vi "Teleop.vi"(10 "Match Info":T1={"Autonomous Elapsed Seconds"=0.0, "TeleOp Elapsed Seconds"=0.0, "Disabled Elapsed Seconds"=0.0, "Visited Autonomous"=FALSE, "Visited TeleOp"=FALSE, "Visited Disabled"=FALSE, "Autonomous Settings"={"Autonomous Style"=enum."Independent", "VI Refnum"=refnum}}, 11 "Call Context":T2) -> ()   [LabVIEW 2015]
doc: "This VI is called for each TeleOp packet received from the DS where the robot is not disabled. It is often used to read from the joysticks and update I/O or to update setpoints for timed control loops. It should complete and return within 20 milliseconds or it may miss DS packets."
uses:
  <vilib>/Rock Robotics/WPI/DriverStation/WPI_DriverStationDerivedRobotMode.ctl
  <vilib>/Rock Robotics/WPI/DriverStation/WPI_DriverStationMatch Info.ctl
  <vilib>/Rock Robotics/WPI/Solenoid/WPI_SolenoidValue.ctl
  <vilib>/Rock Robotics/Network Tables/NT Read Boolean.vi
  <vilib>/Rock Robotics/Network Tables/NT Read Number.vi
  <vilib>/Rock Robotics/WPI/Utilities/WPI_GetSetVariantRefNum.vi
  <vilib>/Rock Robotics/WPI/Solenoid/WPI_SolenoidSetEnum.vi
  <vilib>/addons/control/pid/NI_PID_pid.lvlib
  <vilib>/addons/control/pid/pid.llb/PID (DBL).vi
panel:
  in  "Numeric":dbl
  out "Encodeur gauche min":dbl
  out "Encodeur gauche max":dbl
  out "Encodeur droit max":dbl
  out "Encodeur droit min":dbl
  out "Sample Slider 0":dbl(slide) scale=0.0..5.0
  out "Sample Boolean 1":bool
  out "Sample Boolean 0":bool
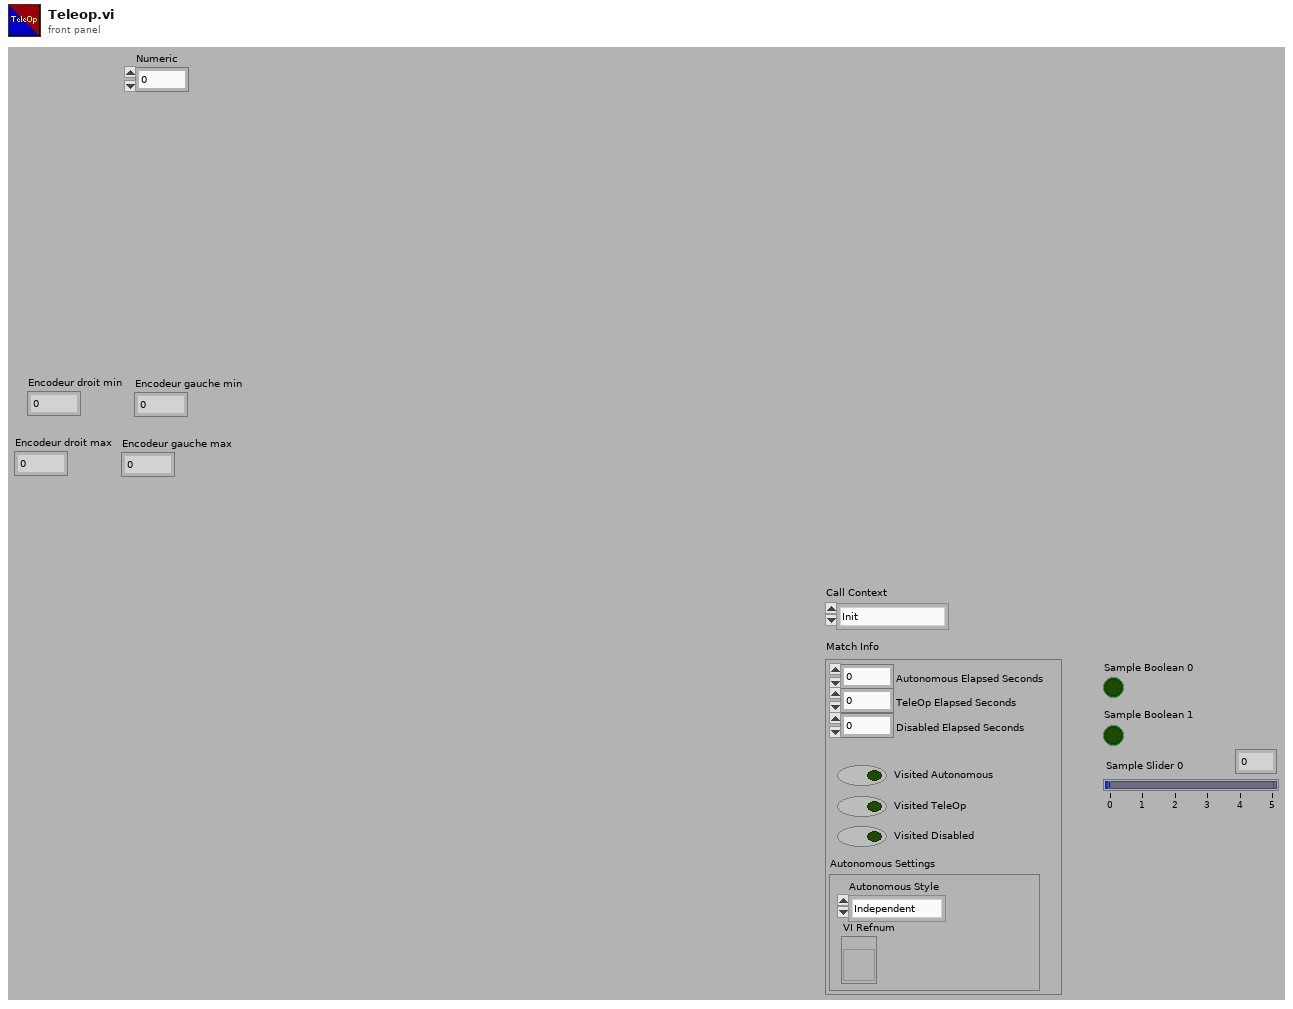
[diagram p1: front panel]
types:
  T1 = typedef "WPI_DriverStationMatch Info.ctl" = cluster{"Autonomous Elapsed Seconds":dbl, "TeleOp Elapsed Seconds":dbl, "Disabled Elapsed Seconds":dbl, "Visited Autonomous":bool, "Visited TeleOp":bool, "Visited Disabled":bool, "Autonomous Settings":cluster{"Autonomous Style":enum16{"Iterative", "Independent"}, "VI Refnum":refnum<vi>}}
  T2 = typedef "WPI_DriverStationDerivedRobotMode.ctl" = enum16{"Init", "Execute", "Stop"}
  T3 = typedef "WPI_JoystickDevRef.ctl" = cluster{"Device":T4}
  T4 = typedef "WPI_JoystickDeviceEnum.ctl" = enum16{"USB 0", "USB 1", "USB 2", "USB 3", "USB 4", "USB 5"}
  T5 = cluster{"Axes[0]":dbl, "Axes[1]":dbl, "Axes[2]":dbl, "Axes[3]":dbl, "Axes[4]":dbl, "Axes[5]":dbl, "Axes[6]":dbl, "Axes[7]":dbl, "Axes[8]":dbl}
  T6 = cluster{"Buttons[0]":bool, "Buttons[1]":bool, "Buttons[2]":bool, "Buttons[3]":bool, "Buttons[4]":bool, "Buttons[5]":bool, "Buttons[6]":bool, "Buttons[7]":bool, "Buttons[8]":bool}
  T7 = typedef "WPI_EncoderDevRef.ctl" = cluster{"DevStatus":errorcluster, "EncoderIndex":T8, "CounterIndex":T9, "DistancePerCount":dbl, "Decoding Type":T10}
  T8 = typedef "FPGA_EncoderIdx.ctl" = enum8{"Enc 0", "Enc 1", "Enc 2", "Enc 3", "Enc 4", "Enc 5", "Enc 6", "Enc 7", "Invalid"}
  T9 = typedef "FPGA_CounterCtrSystemIndex.ctl" = enum8{"Ctr 0", "Ctr 1", "Ctr 2", "Ctr 3", "Ctr 4", "Ctr 5", "Ctr 6", "Ctr 7", "Invalid"}
  T10 = typedef "WPI_EncoderType.ctl" = enum16{"1x", "2x", "4x"}
  T11 = cluster{"proportional gain (Kc)":dbl, "integral time (Ti, min)":dbl, "derivative time (Td, min)":dbl}
  T12 = typedef "WPI_SolenoidDevRef.ctl" = cluster{"DevStatus":errorcluster, "Pneumatics Control Module":u8, "Forward Solenoid Channel":T13, "Reverse Solenoid Channel":T13}
  T13 = typedef "WPI_SolenoidChannel.ctl" = enum8{"Solenoid 0", "Solenoid 1", "Solenoid 2", "Solenoid 3", "Solenoid 4", "Solenoid 5", "Solenoid 6", "Solenoid 7", "Invalid"}
  T14 = typedef "WPI_SolenoidValue.ctl" = enum16{"Off", "On", "Forward", "Reverse"}
  T15 = typedef "WPI_MotorControlDeviceRef.ctl" = cluster{"DeviceStatus":errorcluster, "Type":T16, "PWM":cluster{"PWM Channel":T17, "DeadBand":T18}, "CAN":cluster{"Device Number":u8, "Control Mode":T19, "Semaphore":T20, "Max Vout":dbl, "TalonSRX Control Mode":T21}, "Invert":bool}
  T16 = typedef "WPI_MotorControlType.ctl" = enum16{"PWM", "CAN", "CANTalonSRX"}
  T17 = typedef "FPGA_DIOPWMChannel.ctl" = enum8{"PWM 0", "PWM 1", "PWM 2", "PWM 3", "PWM 4", "PWM 5", "PWM 6", "PWM 7", "PWM 8", "PWM 9", "PWM MXP 0", "PWM MXP 1", "PWM MXP 2", "PWM MXP 3", "PWM MXP 4", "PWM MXP 5", "PWM MXP 6", "PWM MXP 7", "PWM MXP 8", "PWM MXP 9", "Invalid"}
  T18 = typedef "WPI_PWMDeadband.ctl" = cluster{"Name":string, "maxPositivePwm":i32, "minPositivePwm":i32, "centerPwm":i32, "maxNegativePwm":i32, "minNegativePwm":i32, "angularRange":u16}
  T19 = typedef "WPI_CANJaguar_ControlMode.ctl" = enum8{"Percent VBus", "Current", "Speed", "Position", "Voltage"}
  T20 = typedef "Semaphore RefNum" = refnum<k1>
  T21 = typedef "WPI_CANTalonSRX_APIControlMode.ctl" = enum8{"Percent VBus", "Speed", "Position", "Slave", "Unchanged / Invalid", "Voltage Compensation", "Current", "Motion Profile"}
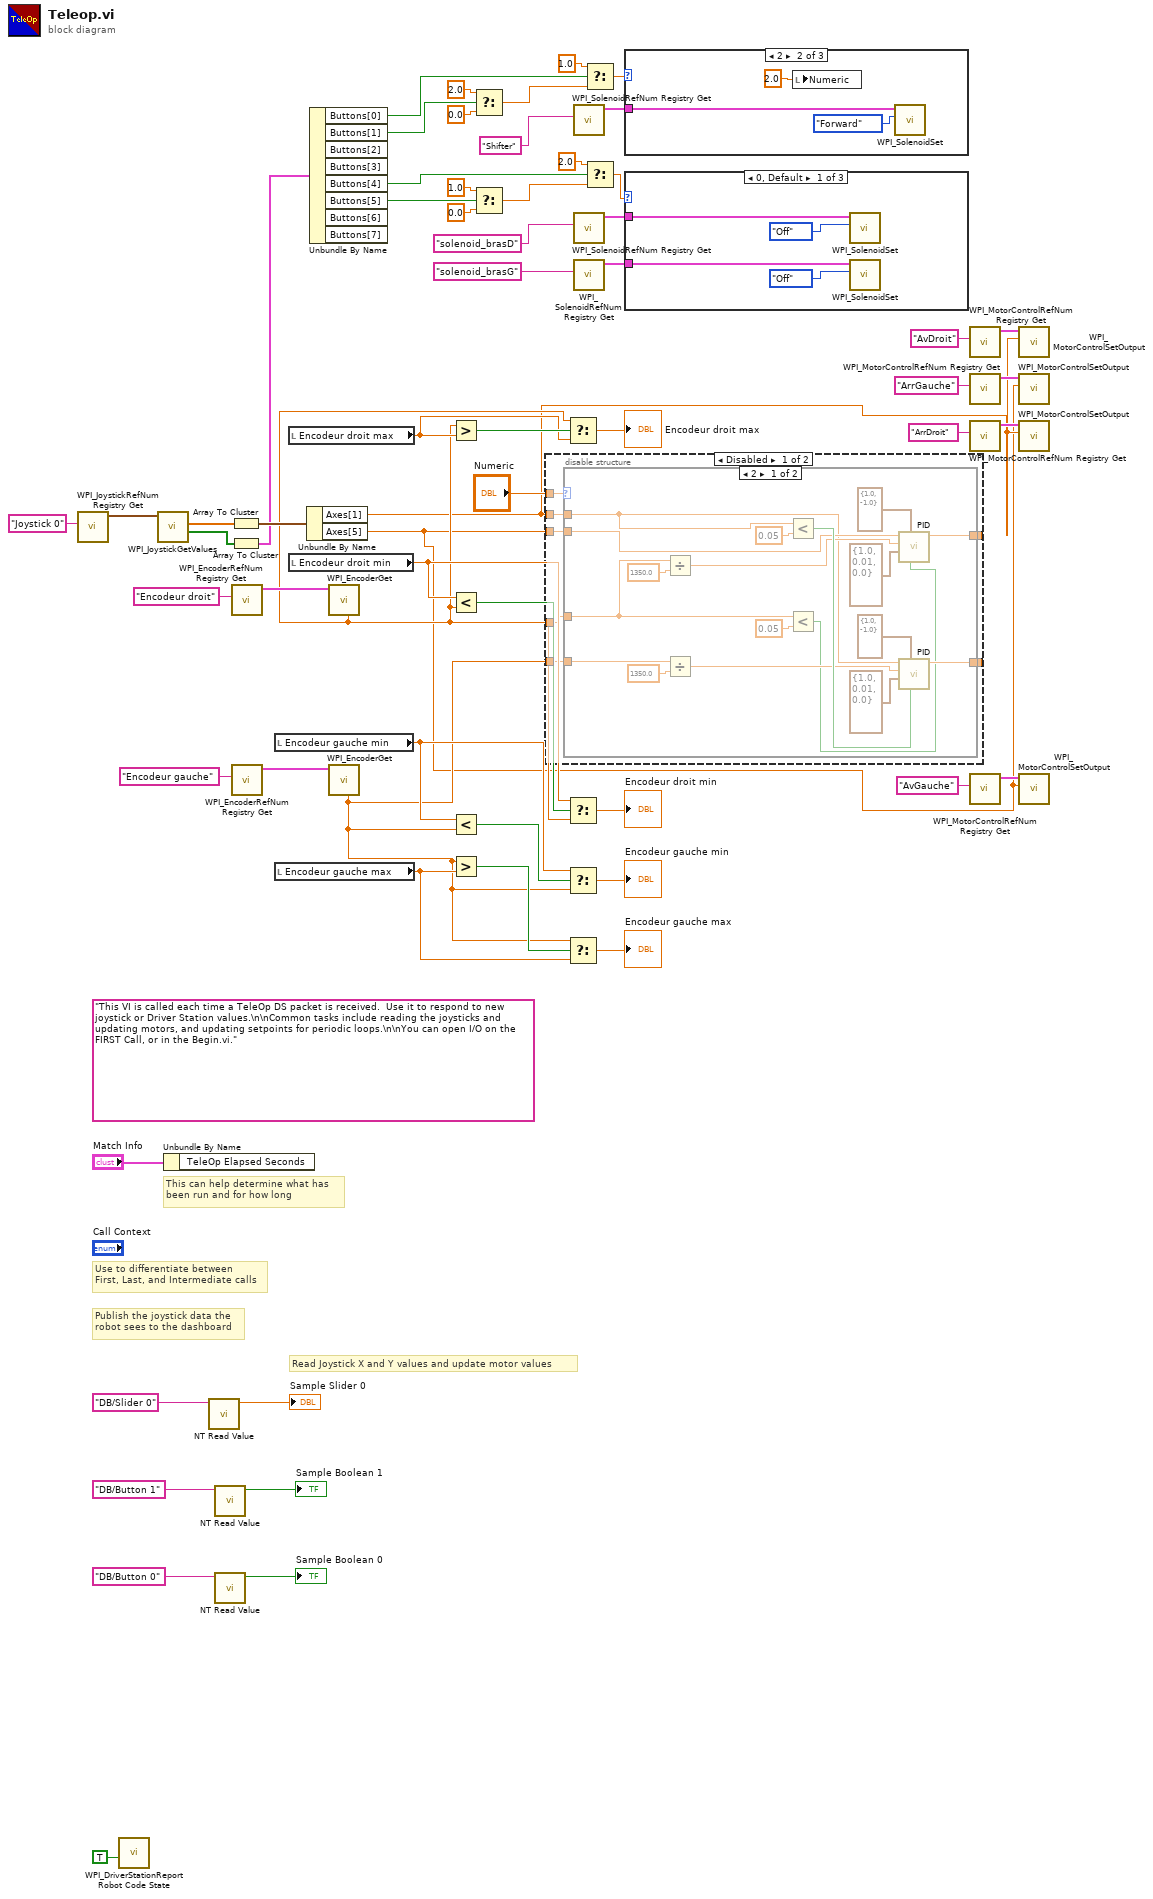
[diagram p0: block diagram]
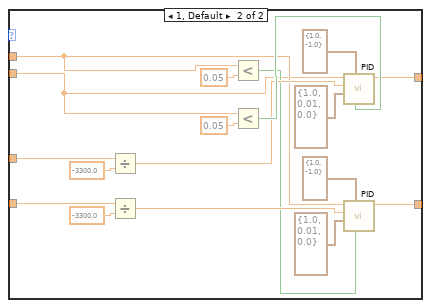
[diagram p2: hidden frame]
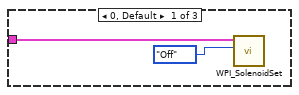
[diagram p4: hidden frame]
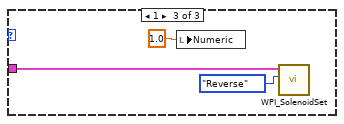
[diagram p5: hidden frame]
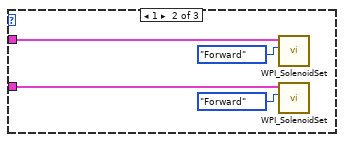
[diagram p6: hidden frame]
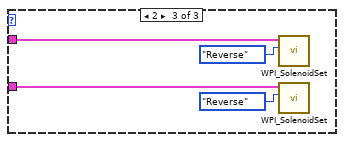
[diagram p7: hidden frame]
diagram:
  (unwired) "This VI is called each time a TeleOp DS packet is received.  Use it to respond to new joystick or Driver Station values.\n\nCommon tasks include reading the joysticks and updating motors, and updating setpoints for periodic loops.\n\nYou can open I/O on the FIRST Call, or in the Begin.vi."
  # "Publish the joystick data the\nrobot sees to the dashboard"
  # "Use to differentiate between\nFirst, Last, and Intermediate calls"
  # "This can help determine what has\nbeen run and for how long"
  # "Read Joystick X and Y values and update motor values"
  n1 = call <vilib>:"WPI_JoystickRefNum Registry Get.vi"("refnum name"="Joystick 0") -> ("JoystickDevRef"=w54:T3)  [unwired: 1 in, 9 out]
  n2 = call <vilib>:"WPI_DriverStationReport Robot Code State.vi"("TeleOp"=TRUE ("Autonomous")) -> ()  [unwired: 10 in, 1 out]
  n3 = call <vilib>:"WPI_JoystickGetValues.vi"("JoystickDevRef"=w54) -> ("Buttons"=w51:bool[], "Axes"=w53:dbl[])  [unwired: 6 in, 3 out]
  n4 = Unbundle By Name("Match Info") -> ()  [unwired: 1 out]
  n5 = call-poly <vilib>:"NT Read Value.vi"("Name"="DB/Slider 0" ("refnum name")) -> ("Numeric"=→"Sample Slider 0":dbl)  [unwired: 9 in, 1 out]
  n6 = call-poly <vilib>:"NT Read Value.vi"("Name"="DB/Button 1" ("refnum name")) -> ("Boolean"=→"Sample Boolean 1":bool)  [unwired: 9 in, 1 out]
  n7 = call-poly <vilib>:"NT Read Value.vi"("Name"="DB/Button 0" ("refnum name")) -> ("Boolean"=→"Sample Boolean 0":bool)  [unwired: 9 in, 1 out]
  n8 = Array To Cluster(array=w53) -> (cluster=w52:T5)
  n9 = Array To Cluster(array=w51) -> (cluster=w9:T6)
  n10 = call <vilib>:"WPI_EncoderRefNum Registry Get.vi"("refnum name"="Encodeur droit") -> ("EncoderDevRef"=w39:T7)  [unwired: 9 in, 1 out]
  n11 = call <vilib>:"WPI_EncoderRefNum Registry Get.vi"("refnum name"="Encodeur gauche") -> ("EncoderDevRef"=w38:T7)  [unwired: 9 in, 1 out]
  n12 = local read "Encodeur gauche min"() -> (w32:dbl)
  n13 = local read "Encodeur gauche max"() -> (w35:dbl)
  n14 = local read "Encodeur droit max"() -> (w30:dbl)
  n15 = local read "Encodeur droit min"() -> (w28:dbl)
  n16 = Unbundle By Name(w52) -> ("Axes[1]"=w2:dbl, "Axes[5]"=w1:dbl)
  n17 = Unbundle By Name(w9) -> ("Buttons[0]"=w8:bool, "Buttons[1]"=w7:bool, "Buttons[4]"=w6:bool, "Buttons[5]"=w5:bool)  [unwired: 4 out]
  n18 = call <vilib>:"WPI_EncoderGet.vi"("EncoderDevRef"=w39) -> ("Rate"=w3:dbl)  [unwired: 5 in, 5 out]
  n19 = call <vilib>:"WPI_EncoderGet.vi"("EncoderDevRef"=w38) -> ("Rate"=w17:dbl)  [unwired: 5 in, 5 out]
  n20 = Greater?(x=w3, y=w30) -> (0:w31:bool)
  n21 = Less?(x=w28, y=w3) -> (x < y?=w29:bool)
  n22 = Less?(x=w32, y=w17) -> (x < y?=w33:bool)
  n23 = Greater?(x=w17, y=w35) -> (0:w36:bool)
  n24 = Select(t=2.0, s=w7, f=0.0) -> (s? t:f=w48:dbl)
  n25 = Select(t=1.0, s=w5, f=0.0) -> (s? t:f=w46:dbl)
  n26 = disable-structure shown="Disabled" {
    disable-tunnel: w17 -> [w70 _]
    disable-tunnel: w1 -> [w69 _]
    disable-tunnel: [w68 _] -> _
    disable-tunnel: w2 -> [w64 _]
    disable-tunnel: [w67 _] -> _
    disable-tunnel: "Numeric" -> [w66 _]
    disable-tunnel: w3 -> [w65 _]
    frame Disabled {
      n27 = case shown="2" w66 {
        tunnel: w64 -> [w72 w90]
        tunnel: [w82 w94] -> w67
        tunnel: w69 -> [w73 w89]
        tunnel: w65 -> [w71 w91]
        tunnel: [w75 w93] -> w68
        tunnel: w70 -> [w74 w92]
        frame 2 {
          n28 = Divide(x=w71, y=1350.0) -> (x/y=w78:dbl)
          n29 = Divide(x=w74, y=1350.0) -> (x/y=w85:dbl)
          n30 = Less?(x=w72, y=0.05) -> (x < y?=w88:bool)
          n31 = Less?(x=w71, y=0.05) -> (x < y?=w81:bool)
          n32 = call-poly <vilib>:"PID.vi"("reinitialize? (F)"=w81, "output range"=cluster{"output high":dbl, "output low":dbl} {"output high"=1.0, "output low"=-1.0}, "PID gains"=T11 {"proportional gain (Kc)"=1.0, "integral time (Ti, min)"=0.01, "derivative time (Td, min)"=0.0}, "process variable"=w78, "setpoint"=w73) -> ("output"=w75:dbl)  [unwired: 5 in, 1 out]
          n33 = call-poly <vilib>:"PID.vi"("reinitialize? (F)"=w88, "output range"=cluster{"output high":dbl, "output low":dbl} {"output high"=1.0, "output low"=-1.0}, "PID gains"=T11 {"proportional gain (Kc)"=1.0, "integral time (Ti, min)"=0.01, "derivative time (Td, min)"=0.0}, "process variable"=w85, "setpoint"=w72) -> ("output"=w82:dbl)  [unwired: 5 in, 1 out]
        }
        frame 1, Default {
          n34 = Divide(x=w91, y=-3300.0) -> (x/y=w98:dbl)
          n35 = Divide(x=w92, y=-3300.0) -> (x/y=w104:dbl)
          n36 = Less?(x=w90, y=0.05) -> (x < y?=w95:bool)
          n37 = Less?(x=w89, y=0.05) -> (x < y?=w101:bool)
          n38 = call-poly <vilib>:"PID.vi"("reinitialize? (F)"=w101, "output range"=cluster{"output high":dbl, "output low":dbl} {"output high"=1.0, "output low"=-1.0}, "PID gains"=T11 {"proportional gain (Kc)"=1.0, "integral time (Ti, min)"=0.01, "derivative time (Td, min)"=0.0}, "process variable"=w98, "setpoint"=w89) -> ("output"=w93:dbl)  [unwired: 5 in, 1 out]
          n39 = call-poly <vilib>:"PID.vi"("reinitialize? (F)"=w95, "output range"=cluster{"output high":dbl, "output low":dbl} {"output high"=1.0, "output low"=-1.0}, "PID gains"=T11 {"proportional gain (Kc)"=1.0, "integral time (Ti, min)"=0.01, "derivative time (Td, min)"=0.0}, "process variable"=w104, "setpoint"=w90) -> ("output"=w94:dbl)  [unwired: 5 in, 1 out]
        }
      }
    }
    frame Enabled {
    }
  }
  n40 = Select(t=w3, s=w31, f=w30) -> (s? t:f=→"Encodeur droit max":dbl)
  n41 = Select(t=w28, s=w29, f=w3) -> (s? t:f=→"Encodeur droit min":dbl)
  n42 = Select(t=w32, s=w33, f=w17) -> (s? t:f=→"Encodeur gauche min":dbl)
  n43 = Select(t=w17, s=w36, f=w35) -> (s? t:f=→"Encodeur gauche max":dbl)
  n44 = call <vilib>:"WPI_SolenoidRefNum Registry Get.vi"("refnum name"="Shifter") -> ("SolenoidDevRef"=w15:T12)  [unwired: 9 in, 1 out]
  n45 = call <vilib>:"WPI_SolenoidRefNum Registry Get.vi"("refnum name"="solenoid_brasD") -> ("SolenoidDevRef"=w10:T12)  [unwired: 9 in, 1 out]
  n46 = call <vilib>:"WPI_SolenoidRefNum Registry Get.vi"("refnum name"="solenoid_brasG") -> ("SolenoidDevRef"=w41:T12)  [unwired: 9 in, 1 out]
  n47 = Select(t=1.0, s=w8, f=w48) -> (s? t:f=w14:dbl)
  n48 = Select(t=2.0, s=w6, f=w46) -> (s? t:f=w42:dbl)
  n49 = case shown="2" w14 {
    tunnel: w15 -> [w108 w111 w113]
    frame 0, Default {
      n50 = call-poly <vilib>:"WPI_SolenoidSet.vi"("Value"=WPI_SolenoidValue."Off", "SolenoidDevRef"=w108) -> ()  [unwired: 8 in, 2 out]
    }
    frame 2 {
      n51 = local write "Numeric"(2.0 ("Numeric")) -> ()
      n52 = call-poly <vilib>:"WPI_SolenoidSet.vi"("Value"=WPI_SolenoidValue."Forward", "SolenoidDevRef"=w111) -> ()  [unwired: 8 in, 2 out]
    }
    frame 1 {
      n53 = local write "Numeric"(1.0 ("Numeric")) -> ()
      n54 = call-poly <vilib>:"WPI_SolenoidSet.vi"("Value"=WPI_SolenoidValue."Reverse", "SolenoidDevRef"=w113) -> ()  [unwired: 8 in, 2 out]
    }
  }
  n55 = case shown="0, Default" w42 {
    tunnel: w41 -> [w117 w122 w125]
    tunnel: w10 -> [w115 w119 w123]
    frame 0, Default {
      n56 = call-poly <vilib>:"WPI_SolenoidSet.vi"("Value"=WPI_SolenoidValue."Off", "SolenoidDevRef"=w115) -> ()  [unwired: 8 in, 2 out]
      n57 = call-poly <vilib>:"WPI_SolenoidSet.vi"("Value"=WPI_SolenoidValue."Off", "SolenoidDevRef"=w117) -> ()  [unwired: 8 in, 2 out]
    }
    frame 1 {
      n58 = call-poly <vilib>:"WPI_SolenoidSet.vi"("Value"=WPI_SolenoidValue."Forward", "SolenoidDevRef"=w119) -> ()  [unwired: 8 in, 2 out]
      n59 = call-poly <vilib>:"WPI_SolenoidSet.vi"("Value"=WPI_SolenoidValue."Forward", "SolenoidDevRef"=w122) -> ()  [unwired: 8 in, 2 out]
    }
    frame 2 {
      n60 = call-poly <vilib>:"WPI_SolenoidSet.vi"("Value"=WPI_SolenoidValue."Reverse", "SolenoidDevRef"=w123) -> ()  [unwired: 8 in, 2 out]
      n61 = call-poly <vilib>:"WPI_SolenoidSet.vi"("Value"=WPI_SolenoidValue."Reverse", "SolenoidDevRef"=w125) -> ()  [unwired: 8 in, 2 out]
    }
  }
  n62 = call <vilib>:"WPI_MotorControlRefNum Registry Get.vi"("refnum name"="AvDroit") -> ("MotorControlDevRef"=w23:T15)  [unwired: 9 in, 1 out]
  n63 = call <vilib>:"WPI_MotorControlRefNum Registry Get.vi"("refnum name"="ArrGauche") -> ("MotorControlDevRef"=w24:T15)  [unwired: 9 in, 1 out]
  n64 = call <vilib>:"WPI_MotorControlRefNum Registry Get.vi"("refnum name"="ArrDroit") -> ("MotorControlDevRef"=w22:T15)  [unwired: 9 in, 1 out]
  n65 = call <vilib>:"WPI_MotorControlRefNum Registry Get.vi"("refnum name"="AvGauche") -> ("MotorControlDevRef"=w25:T15)  [unwired: 9 in, 1 out]
  n66 = call <vilib>:"WPI_MotorControlSetOutput.vi"("Output"=w2, "MotorControlDevRef"=w23) -> ()  [unwired: 7 in, 3 out]
  n67 = call <vilib>:"WPI_MotorControlSetOutput.vi"("Output"=w1, "MotorControlDevRef"=w24) -> ()  [unwired: 7 in, 3 out]
  n68 = call <vilib>:"WPI_MotorControlSetOutput.vi"("Output"=w2, "MotorControlDevRef"=w22) -> ()  [unwired: 7 in, 3 out]
  n69 = call <vilib>:"WPI_MotorControlSetOutput.vi"("Output"=w1, "MotorControlDevRef"=w25) -> ()  [unwired: 7 in, 3 out]
